vi "nanocal generate curvature ellipse V2.vi"(0 "parameter map":map{T4, dbl}(c390), 3 "number of points":i32=20, 5 "2D curvature tensor IN":T1={"curvature Matrix"=[[3.0, 1.0], [1.0, 4.0]], "eigenvs"=[4.618033988749895, 2.381966011250105], "Eigenvectors"=[[-0.8506508083520399+0.0i, -0.5257311121191335+0.0i], [0.5257311121191335+0.0i, -0.8506508083520399+0.0i]], "theta (rad)"=0.5535743588970453, "theta (deg)"=31.717474411461012, "Δs"=[4.618033988749895, 2.381966011250105], "δG/G"=0.5535743588970453, "δs"=[4.618033988749895, 2.381966011250105], "inverse Matrix"=[[3.0, 1.0], [1.0, 4.0]], "noise T"=0.5535743588970453} {"noise T" format="%#_3p"; "inverse Matrix" format="%#_3p"; "δs" format="%#_2p"; "δG/G" format="%#_3p"; "Δs" format="%#_3p"; "theta (deg)" format="%#_3p"; "curvature Matrix" format="%#_3p"; "eigenvs" format="%#_3p"; "Eigenvectors" format="%#_3p"; "theta (rad)" format="%#_3p"}, 9 "data":T5={"dz/dω  (sec/rad)"=[], "z "=[1.7183506006211996e-05-0.0001154032788780638i, 1.7124360968751133e-05-0.0001154114779288915i, 1.7049104347380084e-05-0.00011541542942613611i, 1.700437896335042e-05-0.00011541749156201827i, 1.6984579723285106e-05-0.00011542204741013496i, 1.702277369054923e-05-0.00011543195548892015i, 1.713094025845651e-05-0.00011543928112855599i, 1.734249707866828e-05-0.00011543960094139092i, 1.768320429215342e-05-0.0001154245402225022i, 1.8195281152538477e-05-0.00011538335923575508i, 1.8917228661806973e-05-0.00011530288392402138i, 1.9897834564883332e-05-0.00011516640933089982i, 2.154104046962704e-05-0.0001148906117047364i, 2.3247799321765792e-05-0.00011455940834964969i, 2.5364678450551808e-05-0.00011410149936074356i, 2.8645788781885885e-05-0.00011331572480450341i, 3.204749554800641e-05-0.00011242961468546203i, 3.783559691555022e-05-0.00011080033368711338i, 4.245015867332296e-05-0.00010941815048749576i, 4.909131821431355e-05-0.0001073312840925185i, 5.511821898441184e-05-0.00010535829212367013i, 6.178843506022867e-05-0.00010310289174359778i, 7.1079604965352e-05-9.985157907779013e-05i, 7.922304381453334e-05-9.690255343156676e-05i, 8.814778883893872e-05-9.35627973091444e-05i, 9.806709148886077e-05-8.971246458508318e-05i, 0.00011119043245647465-8.437841897470898e-05i, 0.00012253184919712196-7.953180105990741e-05i, 0.00013777724317049346-7.26422052575784e-05i, 0.0001508081004573332-6.638511645494567e-05i, 0.00016547294918783876-5.890291826790314e-05i, 0.00018003847596605868-5.097295421607585e-05i, 0.00019518361086534857-4.2160672625888326e-05i, 0.00021134179818259658-3.207632261667366e-05i, 0.0002372041782935464-1.434566976209705e-05i, 0.00025518143132024254-7.65423157605567e-07i, 0.0002835129702467886+2.297908707067173e-05i, 0.0003060118087631287+4.414715126576145e-05i, 0.00032860772064336976+6.780161699354136e-05i, 0.0003492674091322389+9.188627597766353e-05i, 0.00037498324855458583+0.0001258445655672888i, 0.00040021078021115026+0.00016463936720210011i, 0.00041969942568205823+0.0001996255883353531i, 0.00044367338947118773+0.00025154867300893595i, 0.0004634793607238068+0.0003068834938295352i, 0.00047921028781215815+0.00036805191402776324i, 0.0004880906353641744+0.00042166295770603194i, 0.0004932212623741357+0.0004947057496862386i, 0.000491476456593048+0.0005562791342814882i, 0.000480893803992059+0.0006363872629062725i, 0.0004535995818650303+0.0007373086546111893i, 0.000417087772881063+0.0008226852134031236i, 0.0003564148692854789+0.0009214817173403453i, 0.0003049201646356487+0.0009841224100520793i, 0.00021260191240459413+0.0010684135492785532i, 0.00011714858948470126+0.001130293664798013i, 1.675457544365132e-05+0.0011752384955043165i, -6.8674075405897e-05+0.0012001399159748158i, -0.000156473047607305+0.0012143601357779102i, -0.00026709373934749337+0.0012167952520739987i, -0.0003544271565676041+0.001206585218500233i, -0.00047937600197311275+0.0011721904461218277i, -0.0006086290582260493+0.0011080263068835828i, -0.0007031877411848573+0.0010369948237613604i, -0.0007564526901441745+0.0009845652865779295i, -0.000802489180995596+0.0009292050493656664i, -0.0008414596018105983+0.0008721985101652608i, -0.0008809346482248761+0.0008000538120167723i, -0.0009073902840241921+0.0007382113118499092i, -0.0009264953054508651+0.000680980624166274i, -0.0009405659412141811+0.0006247883223244968i, -0.000951649722530156+0.0005564170049287236i, -0.0009557485581057351+0.0005027508202624884i, -0.0009558464741053665+0.0004515634249715623i, -0.0009509110176922098+0.0003899637122391104i, -0.0009411315169847015+0.00033238768338539245i, -0.0009303400913929496+0.0002890952314710416i, -0.0009171113529290538+0.00024772942260094455i, -0.0009022111527275027+0.00020961974320628598i, -0.0008813746494947608+0.00016554205395646727i, -0.0008581837971946129+0.00012481593212717478i, -0.0008372063466683705+9.328565348151487e-05i, -0.0008165626610594428+6.595676342721183e-05i, -0.0007901155435838691+3.51376371228606e-05i, -0.0007682834352800848+1.2585785624721776e-05i, -0.000746231015527196-7.956667433689733e-06i, -0.0007238798463130141-2.6771164006128246e-05i, -0.0007015567569177018-4.3779400880525094e-05i, -0.000679301954671598-5.9154880569231366e-05i, -0.0006572001413831251-7.301304884663801e-05i, -0.000629855254567978-8.838260380910578e-05i, -0.0006083942229188815-9.917719243438264e-05i, -0.0005768631156754208-0.00011317657292622015i, -0.0005562177438951648-0.00012121832857134644i, -0.0005359092039599222-0.00012831021292074535i, -0.0005145186443378148-0.00013494179211461784i, -0.0004951602053444319-0.00014023403510992087i, -0.00047624970229075174-0.00014478034103386663i, -0.0004577401041527736-0.00014865456703421655i, -0.00043519037796120065-0.00015262867452433312i], "ω (rad/sec)"=[32012.991918577427, 32390.261658505893, 32466.39798177853, 32499.14340521798, 32517.39286113775, 32529.046092051318, 32537.14525712326, 32543.111142615544, 32547.696343954158, 32551.33675949651, 32554.302325209504, 32556.769142360055, 32558.856995237307, 32560.650202739795, 32562.209843476354, 32563.58125099723, 32564.7987833122, 32565.88895894197, 32566.872575330308, 32567.766175404246, 32568.583086316496, 32569.334166794306, 32570.02835688638, 32570.673085530187, 32571.274580490695, 32571.838104118455, 32572.36813539066, 32572.868514009202, 32573.342552524307, 32573.793126289274, 32574.222746575288, 32574.633618125405, 32575.027687968828, 32575.40668442971, 32575.772149741057, 32576.12546690325, 32576.467883345118, 32576.800529469096, 32577.124435064776, 32577.440543590797, 32577.749724325146, 32578.052781957467, 32578.35046682089, 32578.643482565894, 32578.932492128843, 32579.218126471686, 32579.500987779396, 32579.781656707495, 32580.06069600583, 32580.338656060805, 32580.616078519142, 32580.89350097748, 32581.171461032456, 32581.45050033079, 32581.73116925889, 32582.0140305666, 32582.29966469628, 32582.58867447239, 32582.88169000423, 32583.179375080817, 32583.48243271314, 32583.791613234323, 32584.10772197351, 32584.43162756919, 32584.764273480003, 32585.106690135035, 32585.460007297228, 32585.825472395412, 32586.204468856296, 32586.59853891288, 32587.009410462997, 32587.439030535847, 32587.889604513977, 32588.363642815923, 32588.86402143446, 32589.39405291983, 32589.957576334426, 32590.559071508098, 32591.203800151903, 32591.897990030815, 32592.64907072179, 32593.46598163404, 32594.359581707977, 32595.343197883154, 32596.433373726086, 32597.650906041054, 32599.022313348767, 32600.58195429849, 32602.375161800977, 32604.46301467823, 32606.929831615616, 32609.895397541775, 32613.535812870963, 32618.12101442274, 32624.086899701866, 32632.186064986967, 32643.839295900536, 32662.088751820305, 32694.834175046595, 32770.97049853239]}, 11 "newton parameters":T6={"newton action"=enum."onlygrads", "weighting"=enum."dω √(|dz/dω|)", "PID-P"=0.009761510697263134, "PID-I"=5} {"PID-P" scale=1e-09..1.0 scale format="%#_3p"}, 12 "radius factor":dbl, 14 "ellipse factor":dbl) -> (4 "parameter map OUT":map{T4, dbl}(c390), 6 "2D curvature tensor OUT":T1={"curvature Matrix"=[[3.0, 1.0], [1.0, 4.0]], "eigenvs"=[4.618033988749895, 2.381966011250105], "Eigenvectors"=[[-0.8506508083520399+0.0i, -0.5257311121191335+0.0i], [0.5257311121191335+0.0i, -0.8506508083520399+0.0i]], "theta (rad)"=0.5535743588970453, "theta (deg)"=31.717474411461012, "Δs"=[4.618033988749895, 2.381966011250105], "δG/G"=0.5535743588970453, "δs"=[4.618033988749895, 2.381966011250105], "inverse Matrix"=[[3.0, 1.0], [1.0, 4.0]], "noise T"=0.5535743588970453} {"noise T" format="%#_3p"; "inverse Matrix" format="%#_3p"; "δs" format="%#_2p"; "δG/G" format="%#_3p"; "Δs" format="%#_3p"; "theta (deg)" format="%#_3p"; "curvature Matrix" format="%#_3p"; "eigenvs" format="%#_3p"; "Eigenvectors" format="%#_3p"; "theta (rad)" format="%#_3p"}, 8 "z out":dbl format="%0.2f", 10 "x OUT":dbl[](array[numeric]), 15 "y OUT":dbl[](array[numeric]))   [LabVIEW 2020]
uses:
  3-lorentzian-parameters.ctl
  nanocal -- gradient descent -- parameters.ctl
  3-lorentzian-heat-response action.ctl
  nanocal-goodness-weighting-strategy.ctl
  nanocal -- gradient descent-- data.ctl
  2D curvature tensor.ctl
  <vilib>/Analysis/Matrix/Datatypes/RealMatrix.ctl
  <vilib>/Analysis/Matrix/Datatypes/ComplexMatrix.ctl
  2D curvature tensor actions.ctl
  array of vectors -- algebra.ctl
  array -- fit control .ctl
  nanocal -- gradient descent -- action.ctl
  <vilib>/Analysis/baseanly.llb/Mean (DBL).vi
  generate linear region.vi
  <vilib>/Analysis/baseanly.llb/Inverse Matrix.vi
  <vilib>/Analysis/baseanly.llb/Real Inverse Matrix.vi
  <vilib>/Analysis/7linalg.llb/Eigenvalues and Vectors.vi
  <vilib>/Analysis/7linalg.llb/Real Eigenvalues and Vectors.vi
  <vilib>/Analysis/NI_AALBase.lvlib
  <vilib>/Analysis/Matrix/NI_Matrix.lvlib
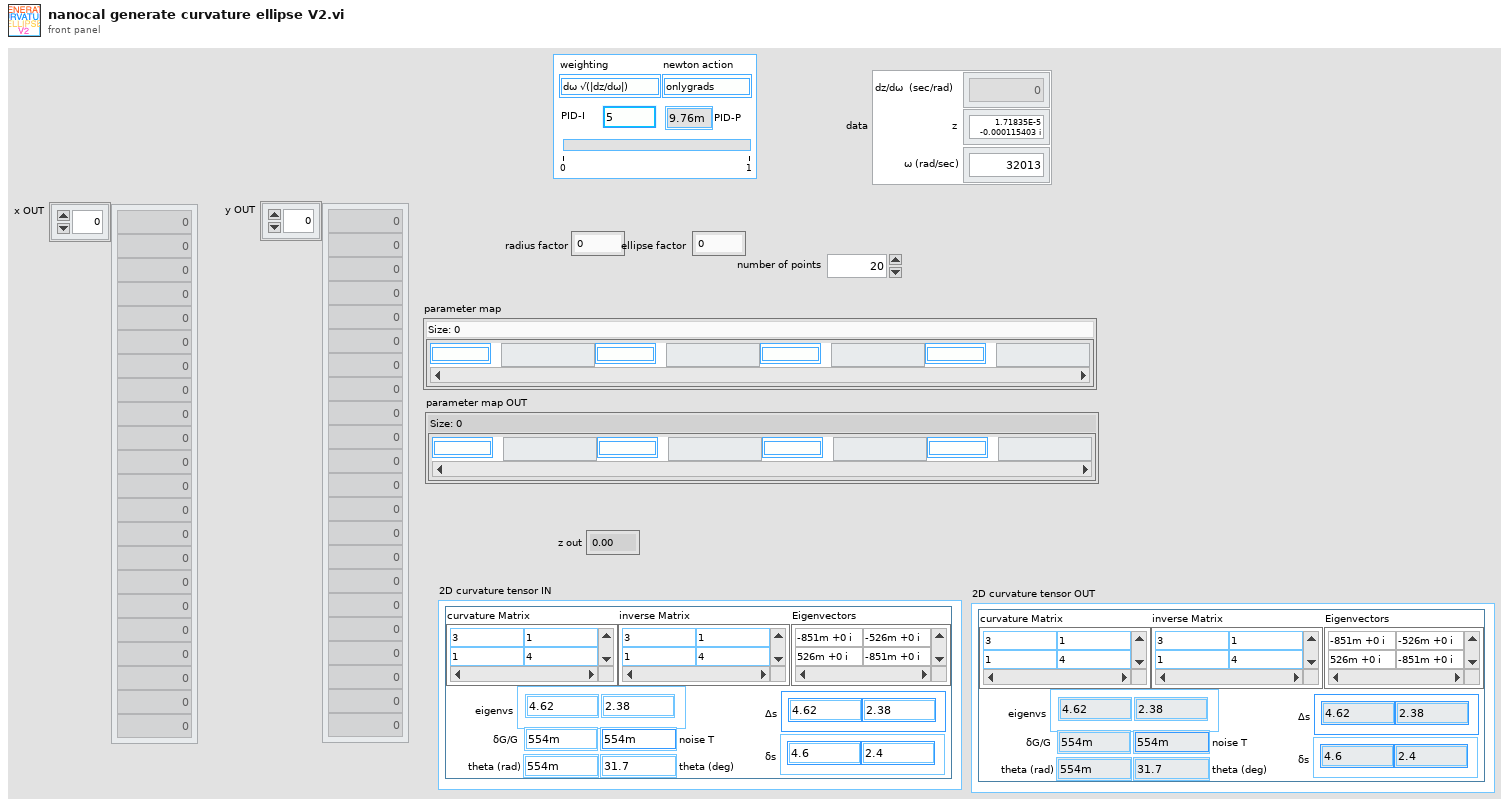
[diagram p1: front panel]
types:
  T1 = typedef "2D curvature tensor.ctl" = cluster{"curvature Matrix":T2, "eigenvs":dbl[], "Eigenvectors":T3, "theta (rad)":dbl, "theta (deg)":dbl, "Δs":dbl[], "δG/G":dbl, "δs":dbl[], "inverse Matrix":T2, "noise T":dbl}
  T2 = typedef "NI_Matrix.lvlib/RealMatrix.ctl" = dbl[][]
  T3 = typedef "NI_Matrix.lvlib/ComplexMatrix.ctl" = cdb[][]
  T4 = typedef "3-lorentzian-parameters.ctl" = enum16{"ζ", "τ1", "τS", "τN", "τC", "κ0", "m1", "m2", "m3", "T (K)", "B (T)", "θ (deg)", "side (S|R)", "set of (B|T)", "Re(offset)", "Im(offset)", "στ1", "στ1-", "στ1+", "στS", "στS-", "στS+"}
  T5 = typedef "nanocal -- gradient descent-- data.ctl" = cluster{"dz/dω  (sec/rad)":cdb[], "z ":cdb[], "ω (rad/sec)":dbl[]}
  T6 = typedef "nanocal -- gradient descent -- parameters.ctl" = cluster{"newton action":T7, "weighting":T8, "PID-P":dbl, "PID-I":i32}
  T7 = typedef "3-lorentzian-heat-response action.ctl" = enum16{"calc R", "create string", "calc m1m2m3", "dζ", "dT1", "dτS", "dτN", "dτC", "d-all", "dκ0", "T(K)", "m1", "m2", "m3", "parse string", "θ (deg)", "B (T)", "onlygrads", "newton", "create emty string"}
  T8 = typedef "nanocal-goodness-weighting-strategy.ctl" = enum16{"dω", "dω √(|dz/dω|)", "dω |dz/dω|", "phase", "andreas", "sum"}
  T9 = typedef "2D curvature tensor actions.ctl" = enum16{"eigensystem", "sigma", "set matrix", "inverse"}
  T10 = typedef "array of vectors -- algebra.ctl" = enum16{"shift", "rotate", "scale", "multiply", "expectation"}
  T11 = typedef "array -- fit control .ctl" = enum16{"fit", "calc", "check", "init"}
  T12 = typedef "nanocal -- gradient descent -- action.ctl" = enum16{"init", "step", "peek"}
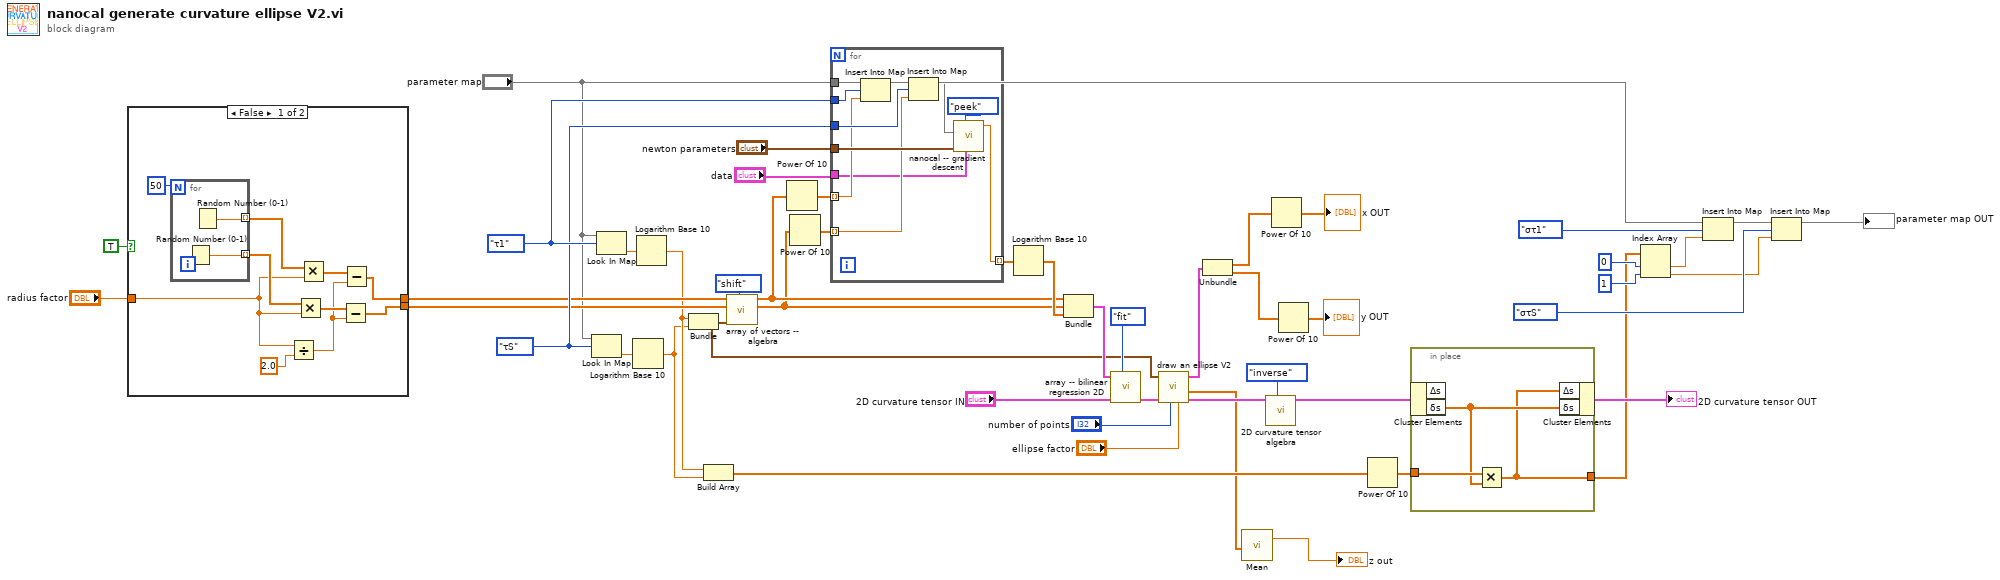
[diagram p0: block diagram]
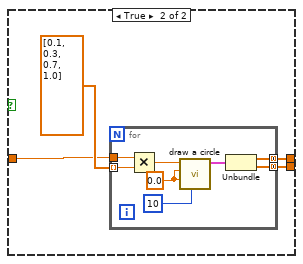
[diagram p2: hidden frame]
diagram:
  w48 = 3-lorentzian-parameters."τS" ("two")
  w49 = 3-lorentzian-parameters."τ1" ("two")
  n1 = case shown="False" TRUE {
    tunnel: [w52 w65] -> w31
    tunnel: [w51 w64] -> w30
    tunnel: "radius factor" -> [w56 w62]
    frame False {
      n2 = for {
        N: 50 -> [_]
        tunnel: [w61] -> w58 mode=indexing
        tunnel: [w60] -> w59 mode=indexing
        n3 = Random Number (0-1)() -> (number: 0 to 1=w60:dbl)
        n4 = Random Number (0-1)() -> (number: 0 to 1=w61:dbl)
      }
      n5 = Divide(x=w56, y=2.0) -> (x/y=w50:dbl)
      n6 = Multiply(x=w59, y=w56) -> (x*y=w53:dbl[])
      n7 = Multiply(x=w58, y=w56) -> (x*y=w54:dbl[])
      n8 = Subtract(x=w53, y=w50) -> (x-y=w51:dbl[])
      n9 = Subtract(x=w54, y=w50) -> (x-y=w52:dbl[])
    }
    frame True {
      n10 = for {
        tunnel: w62 -> [w68]
        tunnel: [w70] -> w65 mode=concatenating
        tunnel: [w69] -> w64 mode=concatenating
        tunnel: dbl[] [0.1, 0.3, 0.7, 1.0] -> [w66] mode=indexing
        w71 = 0.0 ("center x")
        n11 = Multiply(x=w68, y=w66) -> (x*y=w67:dbl)
        n12 = call "draw a circle.vi"("number of points"=10, "center Y"=w71, "center x"=w71, "radius"=w67) -> ("output cluster"=w72:cluster{dbl[], dbl[]})  [unwired: 7 in]
        n13 = Unbundle(w72) -> (w70:dbl[], w69:dbl[])
      }
    }
  }
  n14 = Look In Map(map="parameter map", key=w48) -> (value=w15:dbl)  [unwired: 1 in, 1 out]
  n15 = Look In Map(map="parameter map", key=w49) -> (value=w16:dbl)  [unwired: 1 in, 1 out]
  n16 = Logarithm Base 10(1:w15) -> (0:w13:dbl)
  n17 = Logarithm Base 10(1:w16) -> (0:w14:dbl)
  n18 = Bundle(w14, w13) -> (w17:cluster{dbl, dbl})  [unwired: 1 in]
  n19 = Build Array(w14, w13) -> (w12:dbl[])
  n20 = call "array of vectors -- algebra.vi"("Enum"=array_of_vectors_--_algebra."shift", "vec IN"=w17, "y IN"=w30, "x IN"=w31) -> ("y IOUT"=w28:dbl[], "x  OUT"=w29:dbl[])  [unwired: 5 in, 1 out]
  n21 = Power Of 10(x=w29) -> (10^x=w41:dbl[])
  n22 = Power Of 10(x=w28) -> (10^x=w40:dbl[])
  n23 = for {
    tunnel: w49 -> [w75]
    tunnel: w48 -> [w83]
    tunnel: w41 -> [w77] mode=indexing
    tunnel: w40 -> [w76] mode=indexing
    tunnel: "newton parameters" -> [w81]
    tunnel: "parameter map" -> [w79]
    tunnel: [w78] -> w46 mode=indexing
    tunnel: "data" -> [w74]
    n24 = Insert Into Map(map in=w79, key=w75, value=w77) -> (map out=w84:map{T4, dbl})  [unwired: 2 out]
    n25 = Insert Into Map(map in=w84, key=w83, value=w76) -> (map out=w80:map{T4, dbl})  [unwired: 2 out]
    n26 = call "nanocal -- gradient descent.vi"("data"=w74, "action"=nanocal_--_gradient_descent_--_action."peek", "newton pars"=w81, "parameter Map IN"=w80) -> ("goodness OUT"=w78:dbl)  [unwired: 3 in, 4 out]
  }
  n27 = Logarithm Base 10(1:w46) -> (0:w45:dbl[])
  n28 = Bundle("x  OUT"=w29, "y IOUT"=w28, w45) -> (w43:cluster{"x  OUT":dbl[], "y IOUT":dbl[], dbl[]})  [unwired: 1 in]
  n29 = call "array -- bilinear regression 2D.vi"("action"=array_--_fit_control_."fit", "2D curvature tensor IN"="2D curvature tensor IN", "xyz IN"=w43) -> ("2D curvature tensor OUT"=w7:T1)  [unwired: 5 in, 3 out]
  n30 = call "draw an ellipse V2.vi"("ellipse factor"="ellipse factor", "number of points"="number of points", "2D curvature tensor IN"=w7, "center IN"=w17) -> ("2D curvature tensor OUT"=w19:T1, "z out"=w2:dbl[], "ellipse OUT"=w37:cluster{"Array":dbl[], "Array":dbl[]})  [unwired: 4 in, 1 out]
  n31 = Unbundle(w37) -> ("Array"=w25:dbl[], "Array"=w24:dbl[])
  n32 = call-poly <vilib>:"Mean.vi"("X"=w2) -> ("mean"=→"z out":dbl)  [unwired: 1 out]
  n33 = call "2D curvature tensor algebra.vi"("2D tensor"=2D_curvature_tensor_actions."inverse", "curvature tensor IN"=w19) -> ("curvature tensor OUT"=w11:T1)  [unwired: 8 in, 1 out]
  n34 = Power Of 10(x=w25) -> (10^x=→"x OUT":dbl[])
  n35 = Power Of 10(x=w24) -> (10^x=→"y OUT":dbl[])
  n36 = Power Of 10(x=w12) -> (10^x=w9:dbl[])
  n37 = in-place {
    in-place-border: w9 -> [w87]
    in-place-border: [w85] -> w8
    n38 = in-place-cluster #1(w11) -> ("δs"=w86:dbl[])  [unwired: 1 out]
    n39 = Multiply(x=w87, y=w86) -> (x*y=w85:dbl[])
    n40 = in-place-cluster #1("Δs"=w85, "δs"=w86) -> (→"2D curvature tensor OUT":T1)
  }
  n41 = Index Array(array=w8, index #1=0 ("index"), index #2=1 ("index")) -> (element #1=w21:dbl, element #2=w20:dbl)
  n42 = Insert Into Map(map in="parameter map", key=3-lorentzian-parameters."στ1", value=w21) -> (map out=w36:map{T4, dbl})  [unwired: 2 out]
  n43 = Insert Into Map(map in=w36, key=3-lorentzian-parameters."στS", value=w20) -> (map out=→"parameter map OUT":map{T4, dbl})  [unwired: 2 out]
